vi "Actor Core.vi"(8 "error in":errorcluster, 11 "VisionUI in":refnum<class "VisionUI.lvclass">) -> (0 "error out":errorcluster, 3 "Actor out":refnum<class "Actor.lvclass">)   [LabVIEW 2019, in "VisionUI.lvlib" / "VisionUI.lvclass"]
doc: "(<B>Filename</B>: Actor Framework.lvlib:Actor.lvclass:Actor Core.vi)\n\nReceives messages to the actor, reacts to them, and initiates any error handling that may shut the actor down.\n\nDescendant classes may override this VI to append parallel tasks for the actor to complete while it handles messages. Overrides use the Call Parent Class Method node."
uses:
  VisionUI.lvclass
  C:/Program Files/National Instruments/LabVIEW 2019/vi.lib/ActorFramework/Actor/Actor.lvclass
  <vilib>/ActorFramework/Actor/Actor.lvclass
  <vilib>/userdefined/High Color/IMAQdx.ctl
  <vilib>/ActorFramework/Actor/Actor.lvclass/Actor.ctl
  <vilib>/ActorFramework/Message Enqueuer/Message Enqueuer.lvclass/Message Enqueuer.ctl
  VisionUI.lvclass/VisionUI.ctl
  Vision/Vision Messages/SetROI Msg/SetROI Msg.lvclass/SetROI Msg.ctl
  Vision/Vision Messages/SelectCam Msg/SelectCam Msg.lvclass/SelectCam Msg.ctl
  Vision/Vision Messages/Write Continue Msg/Write Continue Msg.lvclass/Write Continue Msg.ctl
  VisionUI Messages/EnableSave Msg/EnableSave Msg.lvclass/EnableSave Msg.ctl
  ca4c2110-7c99-4ba7-be3f-803697078f68.vi
  <vilib>/ActorFramework/Message Enqueuer/Init from Existing Queue.vi
  <vilib>/ActorFramework/Message Enqueuer/Enqueue.vi
  <vilib>/ActorFramework/Stop Msg/Stop Msg.lvclass
  C:/Program Files/National Instruments/LabVIEW 2019/vi.lib/ActorFramework/Message/Message.lvclass
  Vision/Vision Messages/Snap Msg/Snap Msg.lvclass
  Vision/Vision Messages/SetROI Msg/SetROI Msg.lvclass
  Vision/Vision Messages/SelectCam Msg/SelectCam Msg.lvclass
  Vision/Vision Messages/Save Msg/Save Msg.lvclass
  Vision/Vision Messages/Write Continue Msg/Write Continue Msg.lvclass
  VisionUI Messages/EnableSave Msg/EnableSave Msg.lvclass
  <vilib>/ActorFramework/Message Priority Queue/Priority Enqueue.vi
  <vilib>/JDP Science/JSONtext/JSON text to Variant.vi
  Vision/Vision/Vision.lvclass
  <vilib>/ActorFramework/Message Enqueuer/Message Enqueuer.lvclass
  <vilib>/JDP Science/JSONtext/LVClass Serializer/JSONtext LVClass Serializer.lvclass
panel:
  in  "Capture":bool
  in  "Save?":bool
  in  "SaveROI":bool
  in  "Snap":bool
  in  "Camera":T1
  out "Image":T2(plugin-control)
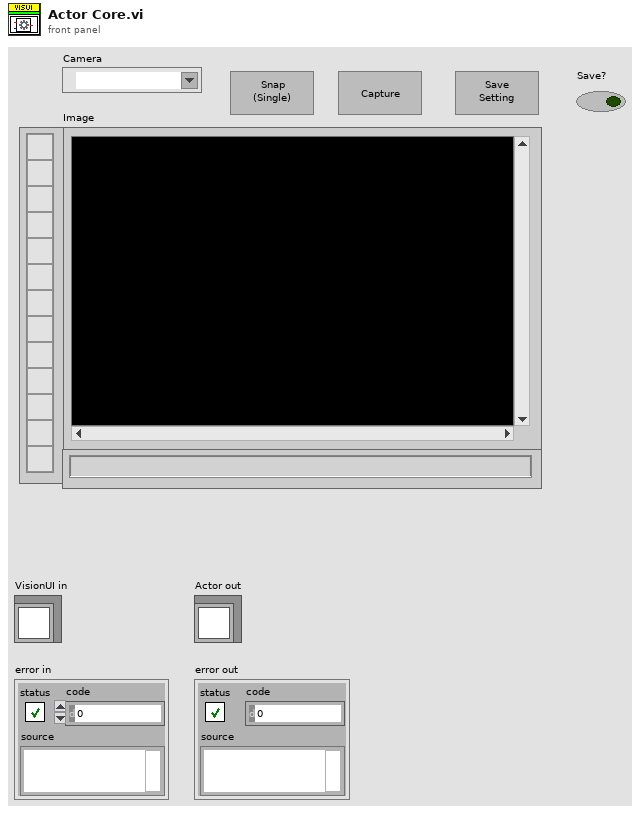
[diagram p1: front panel]
types:
  T1 = typedef "IMAQdx.ctl" = refnum<k21>
  T2 = typedef "IMAQ Image.ctl" = refnum<image>
  T3 = cluster{"stop":refnum<user-event>, "Image":refnum<user-event>, "Extracts":refnum<user-event>, "UI":refnum<user-event>}
  T4 = cluster{"Global Rectangle":i32[], "Contours":cluster{"Contour Type":u32, "ROI Type":u32, "Points":i32[]}[]}
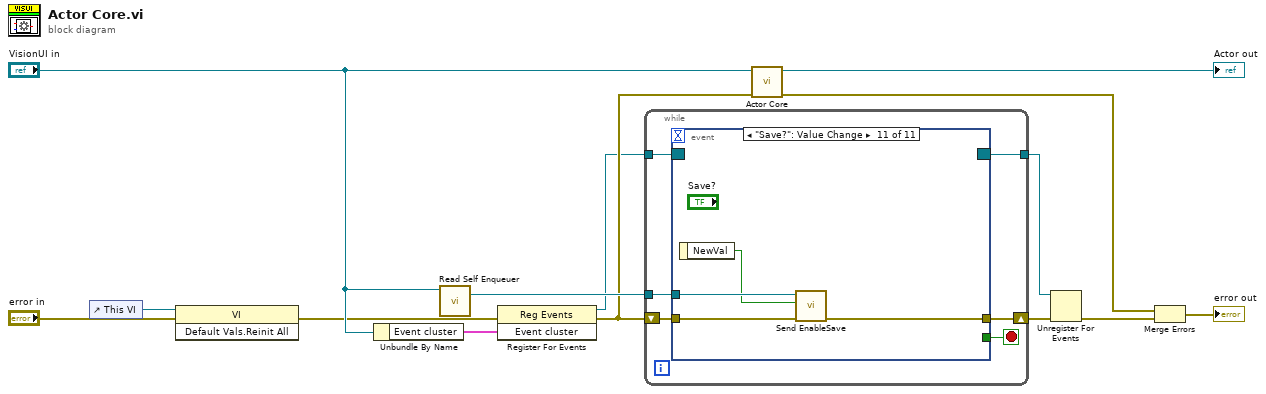
[diagram p0: block diagram]
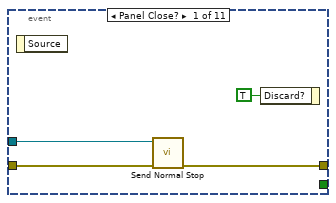
[diagram p2: hidden frame]
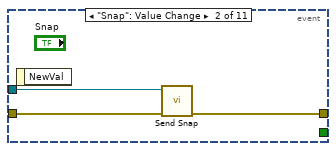
[diagram p3: hidden frame]
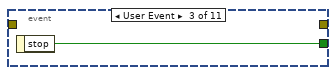
[diagram p4: hidden frame]
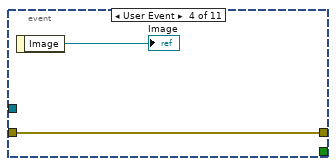
[diagram p5: hidden frame]
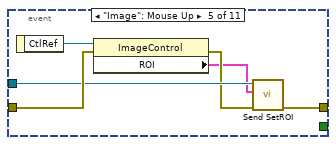
[diagram p6: hidden frame]
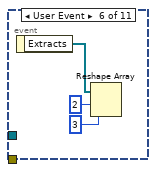
[diagram p7: hidden frame]
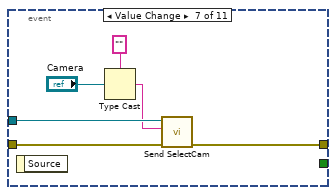
[diagram p8: hidden frame]
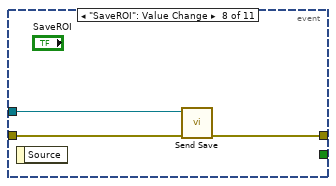
[diagram p9: hidden frame]
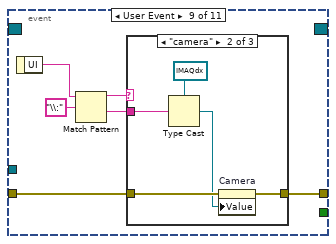
[diagram p10: hidden frame]
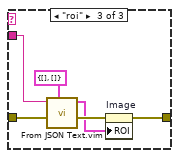
[diagram p12: hidden frame]
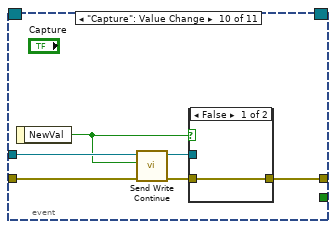
[diagram p13: hidden frame]
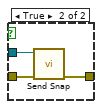
[diagram p14: hidden frame]
diagram:
  n1 = control-ref of="This VI"() -> (w3:refnum<vi>)
  n2 = invoke class="VI" method="Default Vals.Reinit All"(reference=w3, error in="error in") -> (error out=w1:errorcluster)  [unwired: 1 in, 2 out]
  n3 = Unbundle By Name("VisionUI in") -> ("Event cluster"=w12:T3)
  n4 = call <vilib>:"Read Self Enqueuer.vi"("Actor"="VisionUI in") -> ("Self Enqueuer"=w10:refnum<class "Message Enqueuer.lvclass">)  [unwired: 10 in]
  n5 = register-events(error in=w1, w12) -> (reference out=w7:refnum<event-registration>, error out=w9:errorcluster)  [unwired: 1 in]
  n6 = while {
    tunnel: w10 -> [w20]
    shift-right: [w18] -> w5
    shift-left: w9 -> [w19]
    tunnel: w7 -> [w17]
    tunnel: [w16] -> w6
    stop <- w15 stop-if-true
    n7 = event shown="[10] \"Save?\": Value Change" {
      selector: w17 -> [_ _ _ _ _ _ _ _ _ _ _]
      dyn-events: [_ _ _ _ _ _ _ _ _ _ _] -> w16
      timeout: _ -> [_ _ _ _ _ _ _ _ _ _ _]
      tunnel: w20 -> [w23 w27 _ _ w34 _ w45 w47 _ w72 w80]
      tunnel: w19 -> [w22 w26 _ w29 w35 _ w44 w48 w50 w71 w79]
      tunnel: [w21 w25 _ w29 w32 _ w43 w46 w49 w67 w77] -> w18
      tunnel: [_ _ w28 _ _ _ _ _ _ _ _] -> w15
      event Panel Close? {
        n8 = event-data() -> ()  [unwired: 1 in, 1 out]
        n9 = call <vilib>:"Send Normal Stop.vi"("error in (no error)"=w22, "Message Enqueuer"=w23) -> ("error out"=w21:errorcluster)  [unwired: 9 in]
        n10 = event-data("Discard?"=TRUE) -> ()  [unwired: 1 in, 1 out]
      }
      event "Snap": Value Change {
        n11 = event-data() -> ()  [unwired: 1 in, 1 out]
        n12 = call "Send Snap.vi"("error in (no error)"=w26, "Message Enqueuer"=w27) -> ("error out"=w25:errorcluster)  [unwired: 8 in, 1 out]
      }
      event User Event {
        n13 = event-data() -> ("stop"=w28:bool)  [unwired: 1 in]
      }
      event User Event {
        n14 = event-data() -> ("Image"=→"Image":T2)  [unwired: 1 in]
      }
      event "Image": Mouse Up {
        n15 = event-data() -> ("CtlRef"=w36:refnum<vi>)  [unwired: 1 in]
        n16 = property class="ImageControl"(reference=w36, error in=w35) -> (error out=w33:errorcluster, "ROI"=w31:T4)  [unwired: 1 out]
        n17 = call "Send SetROI.vi"("error in (no error)"=w33, "ROI"=w31, "Message Enqueuer"=w34) -> ("error out"=w32:errorcluster)  [unwired: 7 in, 1 out]
      }
      event User Event {
        n18 = event-data() -> ("Extracts"=w37:T2[])  [unwired: 1 in]
        n19 = Reshape Array(w37, 2 ("dimension size"), 3 ("dimension size")) -> ()  [unwired: 1 out]
      }
      event Value Change {
        n20 = event-data() -> ()  [unwired: 1 in, 1 out]
        n21 = Type Cast(type="", x="Camera") -> (*(type *) &x=w40:string)
        n22 = call "Send SelectCam.vi"("error in (no error)"=w44, "Cam Session"=w40, "Message Enqueuer"=w45) -> ("error out"=w43:errorcluster)  [unwired: 7 in, 1 out]
      }
      event "SaveROI": Value Change {
        n23 = event-data() -> ()  [unwired: 1 in, 1 out]
        n24 = call "Send Save.vi"("error in (no error)"=w48, "Message Enqueuer"=w47) -> ("error out"=w46:errorcluster)  [unwired: 8 in, 1 out]
      }
      event User Event {
        n25 = event-data() -> ("UI"=w54:string)  [unwired: 1 in]
        n26 = Match Pattern(string=w54, regular expression="\\:") -> (before substring=w52:string, after substring=w51:string)  [unwired: 1 in, 2 out]
        n27 = case shown="\"camera\"" w52 {
          tunnel: w51 -> [_ w58 w64]
          tunnel: w50 -> [w55 w60 w66]
          tunnel: [w55 w59 w61] -> w49
          frame Default {
          }
          frame "camera" {
            n28 = Type Cast(type=T1 refnum ("Camera"), x=w58) -> (*(type *) &x=w56:T1)
            n29 = property on="Camera" class="IMAQdx (strict)"(error in=w60, "Value"=w56) -> (error out=w59:errorcluster)  [unwired: 1 in, 1 out]
          }
          frame "roi" {
            n30 = call "From JSON Text.vim"("Data Type and Default Value"=T4 {"Global Rectangle"=[], "Contours"=[]} ("ROI"), "error in (no error)"=w66, "JSON"=w64) -> ("error out"=w63:errorcluster, "Data out"=w62:T4)  [unwired: 7 in]
            n31 = property on="Image" class="ImageControl"(error in=w63, "ROI"=w62) -> (error out=w61:errorcluster)  [unwired: 1 in, 1 out]
          }
        }
      }
      event "Capture": Value Change {
        n32 = event-data() -> ("NewVal"=w69:bool)  [unwired: 1 in]
        n33 = call "Send Write Continue.vi"("error in (no error)"=w71, "Continue"=w69, "Message Enqueuer"=w72) -> ("error out"=w70:errorcluster, "Message Enqueuer out"=w68:refnum<class "Message Enqueuer.lvclass">)  [unwired: 7 in]
        n34 = case shown="False" w69 {
          tunnel: w70 -> [w73 w76]
          tunnel: w68 -> [_ w75]
          tunnel: [w73 w74] -> w67
          frame False {
          }
          frame True {
            n35 = call "Send Snap.vi"("error in (no error)"=w76, "Message Enqueuer"=w75) -> ("error out"=w74:errorcluster)  [unwired: 8 in, 1 out]
          }
        }
      }
      event "Save?": Value Change {
        n36 = event-data() -> ("NewVal"=w78:bool)  [unwired: 1 in]
        n37 = call "Send EnableSave.vi"("error in (no error)"=w79, "Save"=w78, "Message Enqueuer"=w80) -> ("error out"=w77:errorcluster)  [unwired: 7 in, 1 out]
      }
    }
  }
  n38 = call-parent "Actor Core.vi"("error in"=w9, "Actor in"="VisionUI in") -> ("error out"=w14:errorcluster, "Actor out"=→"Actor out":refnum<class "Actor.lvclass">)  [unwired: 8 in]
  n39 = Unregister For Events(event registration refnum=w6, error in=w5) -> (error out=w4:errorcluster)
  n40 = Merge Errors(w14, w4) -> (→"error out":errorcluster)
